vi "db status.vi"(0 "para0":dbl, 1 "resetFlg":i32, 5 "op":i32, 7 "pCur":i32, 9 "pHiwtr":i32, 11 "error in (no error)":errorcluster) -> (4 "para0 out":dbl, 6 "function return":i32, 8 "pCur out":i32, 10 "pHiwtr out":i32, 15 "error out":errorcluster)   [LabVIEW 2020, in "sqlite3.lvlib"]
uses:
  sqlite3.lvlib
  errstr.vi
  bin/sqlite3_64.dll
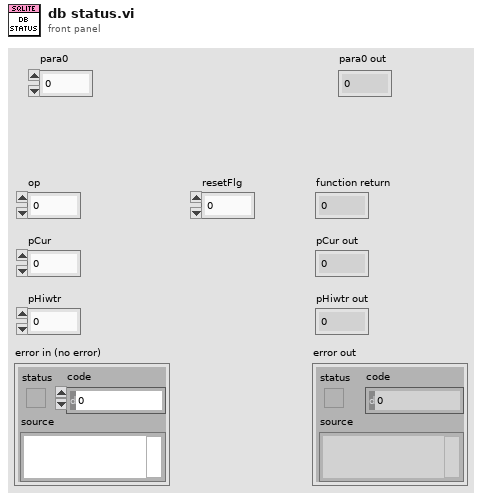
[diagram p1: front panel]
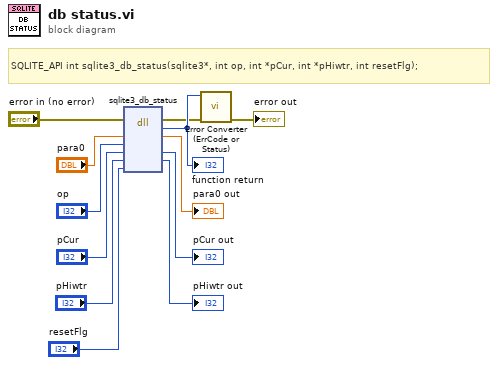
[diagram p0: block diagram]
diagram:
  # "SQLITE_API int sqlite3_db_status(sqlite3*, int op, int *pCur, int *pHiwtr, int resetFlg);"
  n1 = dll-call lib="C:/Users/Fred.Guo/Desktop/Database-configuration/externals/sqlite3/Source/bin/sqlite3_*.*" fn="sqlite3_db_status"(error in="error in (no error)", "para0"="para0", "op"="op", "pCur"="pCur", "pHiwtr"="pHiwtr", "resetFlg"="resetFlg") -> (error out=w2:errorcluster, w12:i32, "para0"=→"para0 out":dbl, "pCur"=→"pCur out":i32, "pHiwtr"=→"pHiwtr out":i32)  [unwired: 4 in, 1 out]
  "function return" <- w12
  n2 = call "Error Converter (ErrCode or Status).vi"("error in (no error)"=w2, "error code"=w12) -> ("error out"=→"error out":errorcluster)  [unwired: 9 in]
